vi "Determine Node Type.vi"(9 "Parent Type":T1, 10 "Refnum in":refnum<k21>) -> (2 "Node Type":T1)   [LabVIEW 2016, in "Synchronised Tag.lvclass"]
uses:
  Synchronised Tag.lvclass
  Controls/Node Type.ctl
  <resource>/objmgr/ni.var.rc
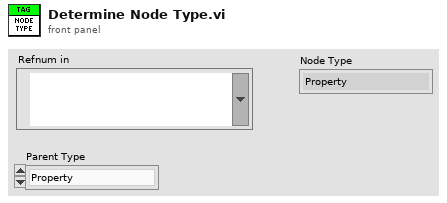
[diagram p1: front panel]
types:
  T1 = typedef "Node Type.ctl" = enum16{"Property", "Item", "Folder"}
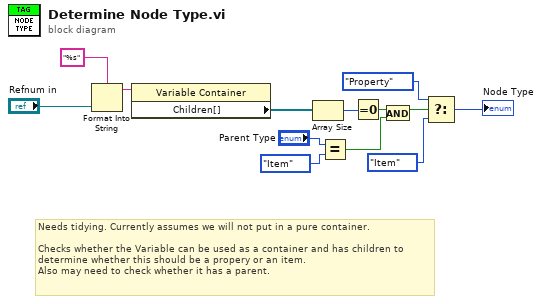
[diagram p0: block diagram]
diagram:
  # "Needs tidying. Currently assumes we will not put in a pure container.\n\nChecks whether the Variable can be used as a container and has children to\ndetermine whether this should be a propery or an item.\nAlso may need to check whether it has a parent."
  n1 = Format Into String(format string="%s", "Refnum in") -> (resulting string=w9:string)  [unwired: 2 in, 1 out]
  n2 = property class="Variable Container"(reference=w9) -> ("Children[]"=w10:refnum<k21>[])  [unwired: 1 in, 2 out]
  n3 = Array Size(array=w10) -> (size(s)=w11:i32)
  n4 = Equal?(x="Parent Type", y=Node_Type."Item" ("Node Type")) -> (x = y?=w1:bool)
  n5 = Equal To 0?(x=w11) -> (x = 0?=w5:bool)
  n6 = And(x=w5, y=w1) -> (x .and. y?=w4:bool)
  n7 = Select(t=Node_Type."Property" ("Node Type"), s=w4, f=Node_Type."Item" ("Node Type")) -> (s? t:f=→"Node Type":T1)
